vi "getAlignmentFromDocument.vi"(8 "error in (no error)":errorcluster, 11 "xwpfParagraph in":refnum<class "xwpfParagraph.lvclass">) -> (0 "error out":errorcluster, 3 "xwpfParagraph out":refnum<class "xwpfParagraph.lvclass">)   [LabVIEW 2017, in "Word_Specific.lvlib" / "xwpfParagraph.lvclass"]
uses:
  xwpfParagraph.lvclass
  xwpfParagraph.lvclass/xwpfParagraph.ctl
  C:/Users/Neo/Desktop/Dev_Tools_BR/LabVIEW_NPOI/lib/NPOI 2.1.1/NPOI.OOXML.dll
  lib/NPOI 2.1.1/NPOI.OOXML.dll
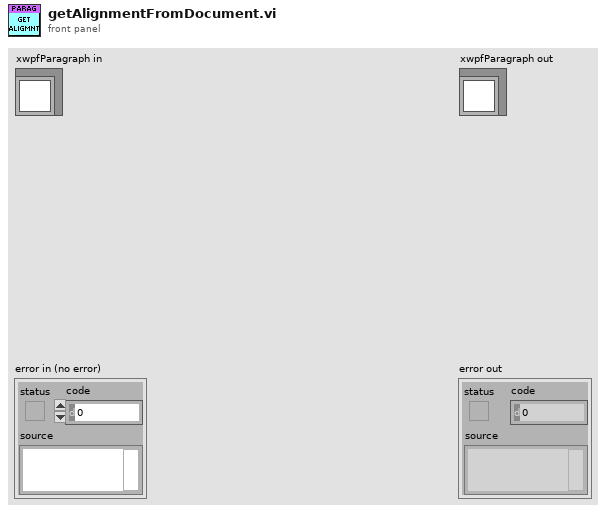
[diagram p1: front panel]
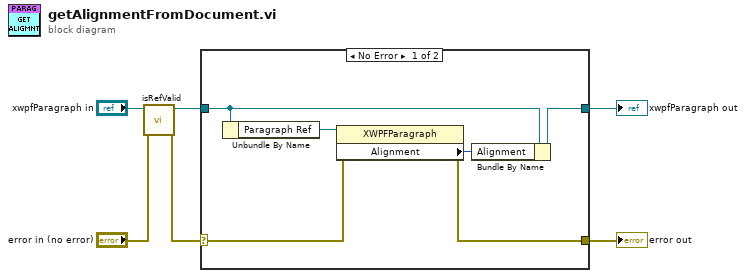
[diagram p0: block diagram]
diagram:
  n1 = call-dynamic "isRefValid.vi"("error in (no error)"="error in (no error)", "xwpfParagraph in"="xwpfParagraph in") -> ("error out"=w1:errorcluster, "xwpfParagraph out"=w3:refnum<class "xwpfParagraph.lvclass">)  [unwired: 8 in]
  n2 = case shown="No Error" w1 {
    selector: w1 -> [w8 w14]
    tunnel: [w7 w14] -> w6
    tunnel: [w10 w13] -> w4
    tunnel: w3 -> [w12 w13]
    frame No Error {
      n3 = Unbundle By Name(w12) -> ("Paragraph Ref"=w11:refnum<k24>)
      n4 = property class="XWPFParagraph"(reference=w11, error in=w8) -> (error out=w7:errorcluster, "Alignment"=w9:i32)  [unwired: 1 out]
      n5 = Bundle By Name(cluster=w12, "Alignment"=w9) -> (w10:refnum<class "xwpfParagraph.lvclass">)
    }
    frame Error {
    }
  }
  "error out" <- w6
  "xwpfParagraph out" <- w4
